vi "Configuration parameter writing.vi"(9 "enable":bool caption="值", 10 "baud rate (9600)":u32(ring)=4800 caption="波特率" items=["1200"=1200, "2400"=2400, "4800"=4800, "9600"=9600, "19200"=19200, "38400"=38400, "115200"=115200], 11 "VISA resource name":refnum<visa-resource-name> caption="串口") -> ()   [LabVIEW 2016, in "AIRMAR WeatherCaster.lvlib"]
uses:
  AIRMAR WeatherCaster.lvlib
  <vilib>/Utility/config.llb/Write Key (String).vi
  <vilib>/Utility/config.llb/Write Key (U32).vi
  <vilib>/Utility/config.llb/Write Key (Boolean).vi
  <vilib>/Utility/config.llb/NI_LVConfig.lvlib
panel:
  out "error out":errorcluster caption="错误输出"
  in  "error in (no error)":errorcluster caption="错误输入（无错误）"
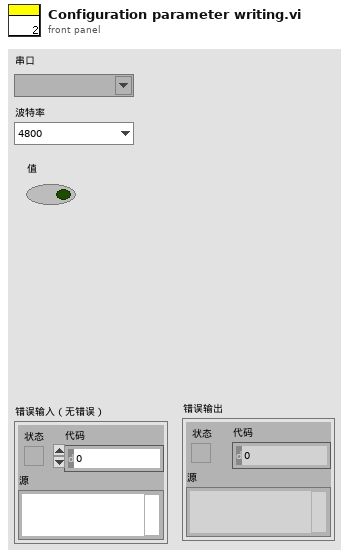
[diagram p1: front panel]
types:
  T1 = typedef "NI_LVConfig.lvlib/Config Data RefNum.ctl" = refnum<k1>
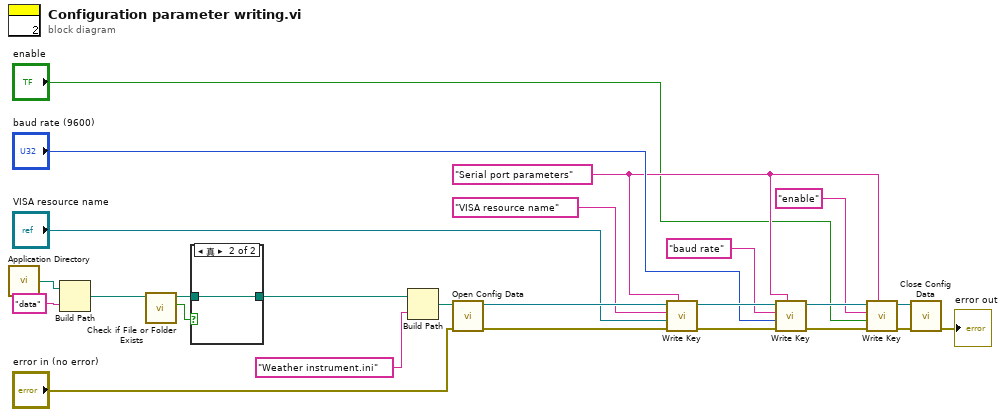
[diagram p0: block diagram]
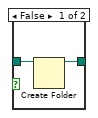
[diagram p2: hidden frame]
diagram:
  w5 = "Serial port parameters" ("section")
  n1 = call <vilib>:"Application Directory.vi"() -> ("Application Directory"=w13:path)
  n2 = Build Path(base path=w13, name or relative path="data" ("名称或相对路径")) -> (appended path=w11:path)
  n3 = call <vilib>:"Check if File or Folder Exists.vi"("path"=w11) -> ("file or folder exists?"=w10:bool, "dup path"=w9:path)  [unwired: 8 in, 1 out]
  n4 = case shown="真" w10 {
    tunnel: w9 -> [w27 w28]
    tunnel: [w26 w28] -> w8
    frame False {
      n5 = Create Folder(path (use dialog)=w27) -> (created path=w26:path)  [unwired: 2 in, 2 out]
    }
    frame True {
    }
  }
  n6 = Build Path(base path=w8, name or relative path="Weather instrument.ini" ("名称或相对路径")) -> (appended path=w23:path)
  n7 = call <vilib>:"Open Config Data.vi"("error in (no error)"="error in (no error)", "configuration file path"=w23) -> ("error out"=w24:errorcluster, "refnum"=w25:T1)  [unwired: 7 in, 1 out]
  n8 = call-poly <vilib>:"Write Key.vi"("section"=w5, "error in (no error)"=w24, "value"="VISA resource name", "key"="VISA resource name", "refnum"=w25) -> ("error out"=w19:errorcluster, "refnum out"=w20:T1)  [unwired: 4 in, 1 out]
  n9 = call-poly <vilib>:"Write Key.vi"("section"=w5, "error in (no error)"=w19, "value"="baud rate (9600)", "key"="baud rate", "refnum"=w20) -> ("error out"=w7:errorcluster, "refnum out"=w6:T1)  [unwired: 4 in, 1 out]
  n10 = call-poly <vilib>:"Write Key.vi"("section"=w5, "error in (no error)"=w7, "value"="enable", "key"="enable", "refnum"=w6) -> ("error out"=w3:errorcluster, "refnum out"=w4:T1)  [unwired: 4 in, 1 out]
  n11 = call <vilib>:"Close Config Data.vi"("error in (no error)"=w3, "refnum"=w4) -> ("error out"=→"error out":errorcluster)  [unwired: 8 in, 1 out]
